vi "Theme Definer UI.vi"() -> ()   [LabVIEW 2021]
doc: "This VI provides a user interface for creating theme style files to output\n\n<b>Code Developed By:</b> +\nDaniel Coons +\nhttps://github.com/danielcoons/tsc-pop-up"
uses:
  Theme/Dialog colors--typedef.ctl
  Theme/Button colors--typedef.ctl
  Theme/message box--typdef.ctl
  <vilib>/picture/picture.llb/imagedata.ctl
  Theme/Theme.lvclass/Theme.ctl
  Popup/PopUp Theme Global.vi
  Theme/Theme.lvclass
  user32.dll
panel:
  in  "Tab Control":enum32{"style file", "material file"}(tab)
  in  "File (.style)":path
  in  "save":bool
  in  "File (.xml)":path
  in  "Theme":u16(ring) items=["Light Theme", "Light Medium Contrast", "Light High Contrast", "Dark Theme", "Dark Medium Contrast", "Dark High Constrast"]
  out "pop-up header":bool
  out "2D Picture":picture
  in  "OK Button":bool
  out "String":string="message input preview"
  in  "Input-string":string="preview"
  in  "Exit":bool
  out "Header":bool
  in  "input":T1={"Text.Font Name"="Segoe UI", "Text.Font Size"=30, "Color"=6579300, "Text.Justification"=enum."Center", "messge color"={"border"=16777215, "fill"=16777215}}
  in  "message font":T1={"Text.Font Name"="Segoe UI", "Text.Font Size"=30, "Color"=6579300, "Text.Justification"=enum."Center", "messge color"={"border"=15790320, "fill"=16777215}}
  in  "button colors":T2={"false color"={"border"=14869218, "fill"=16777215}, "hover color"={"border"=0, "fill"=0}, "press color"={"border"=6579300, "fill"=6579300}, "Boolean Text"=6579300, "Text.Font Name"="Segoe UI", "Text.Font Size"=20, "Bold?"=TRUE, "Itallic?"=FALSE}
  in  "dialog colors":T3={"Header"=11579568, "Background"=15790320, "Picture Background"=16777216}
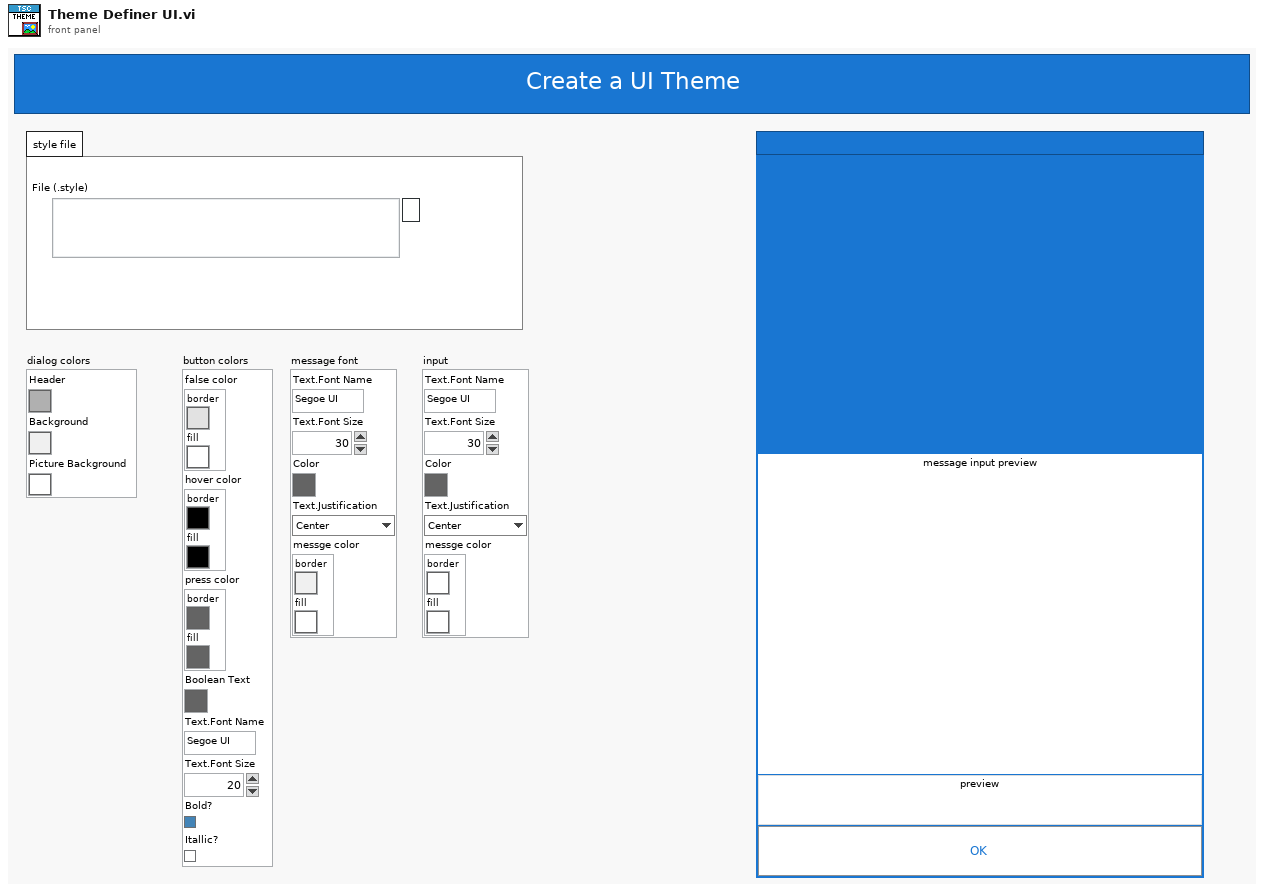
[diagram p1: front panel]
types:
  T1 = typedef "Theme.lvclass/message box--typdef.ctl" = cluster{"Text.Font Name":string, "Text.Font Size":u32, "Color":u32, "Text.Justification":enum16{"Left", "Center", "Right"}, "messge color":cluster{"border":u32, "fill":u32}}
  T2 = typedef "Theme.lvclass/Button colors--typedef.ctl" = cluster{"false color":cluster{"border":u32, "fill":u32}, "hover color":cluster{"border":u32, "fill":u32}, "press color":cluster{"border":u32, "fill":u32}, "Boolean Text":u32, "Text.Font Name":string, "Text.Font Size":u32, "Bold?":bool, "Itallic?":bool}
  T3 = typedef "Theme.lvclass/Dialog colors--typedef.ctl" = cluster{"Header":u32, "Background":u32, "Picture Background":u32}
  T4 = typedef "imagedata.ctl" = cluster{"image type":i32, "image depth":i32, "image":u8[], "mask":u8[], "colors":u32[], "Rectangle":cluster{"left":i16, "top":i16, "right":i16, "bottom":i16}}
  T5 = cluster{"left":i16, "top":i16, "right":i16, "bottom":i16}
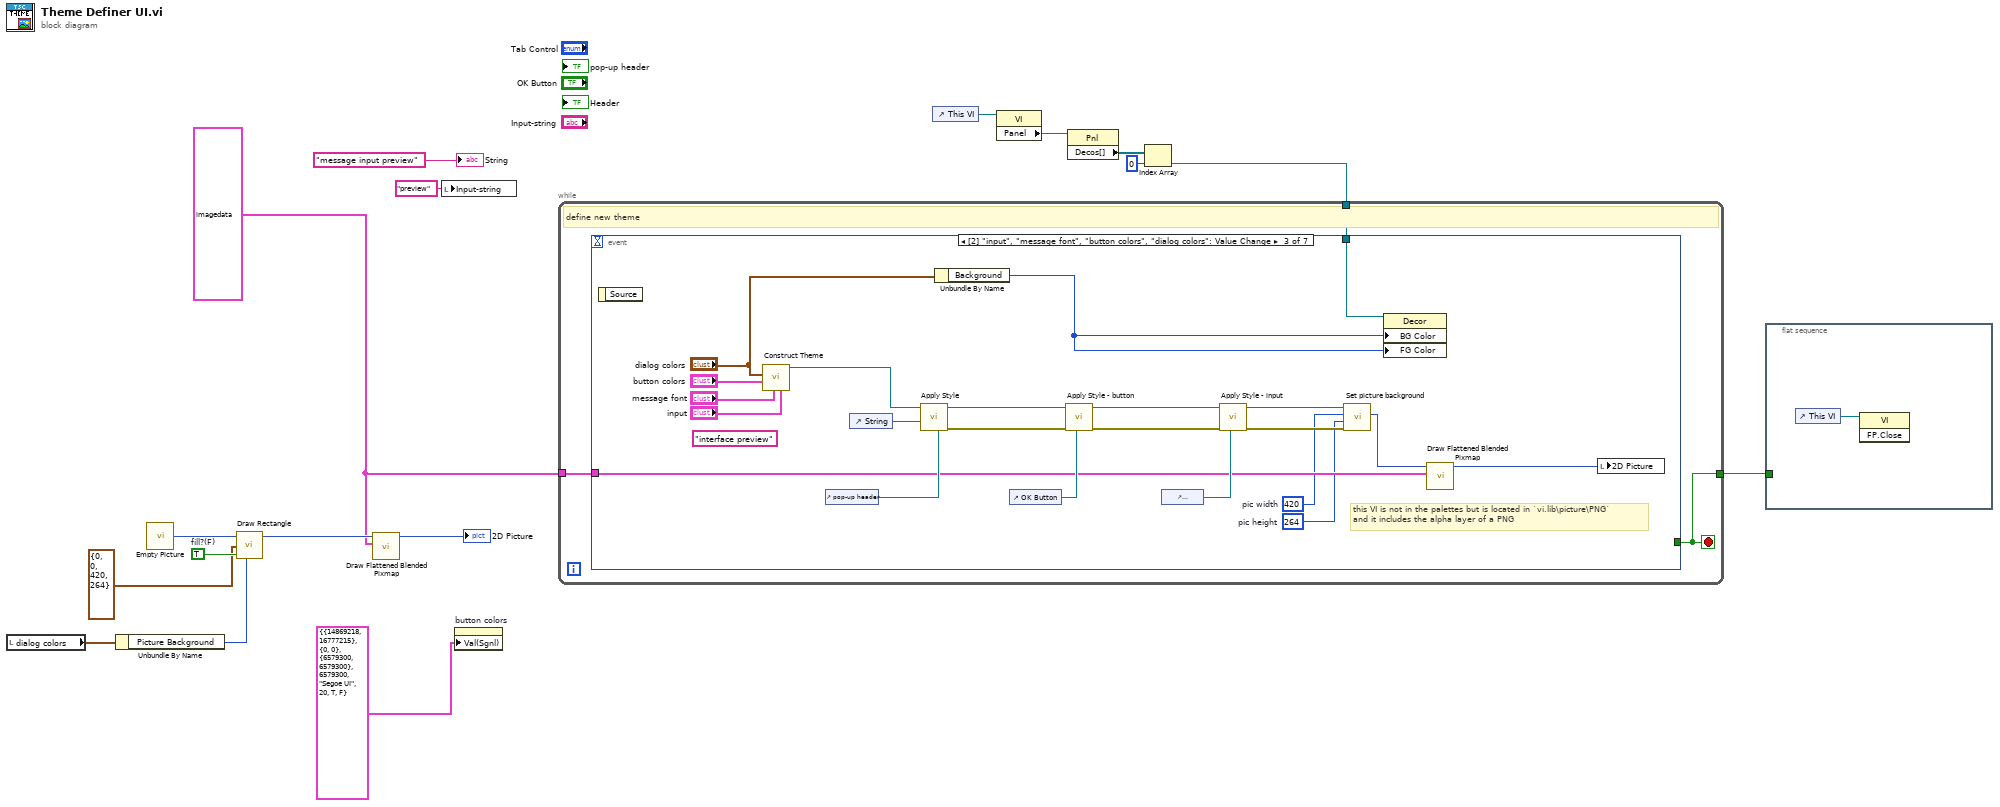
[diagram p0: block diagram]
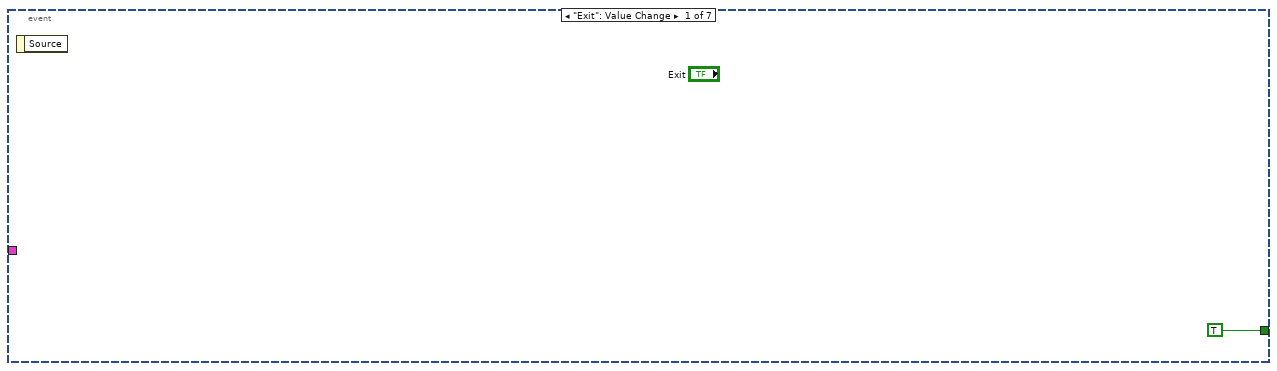
[diagram p2: hidden frame]
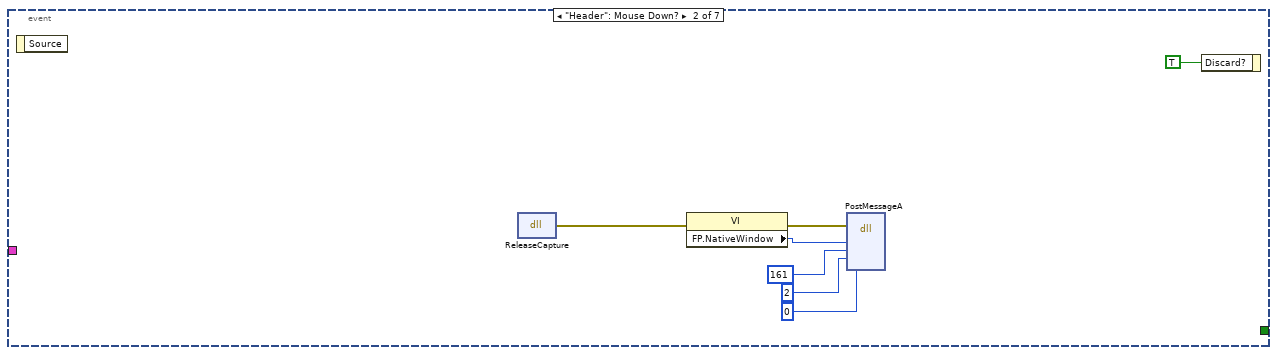
[diagram p3: hidden frame]
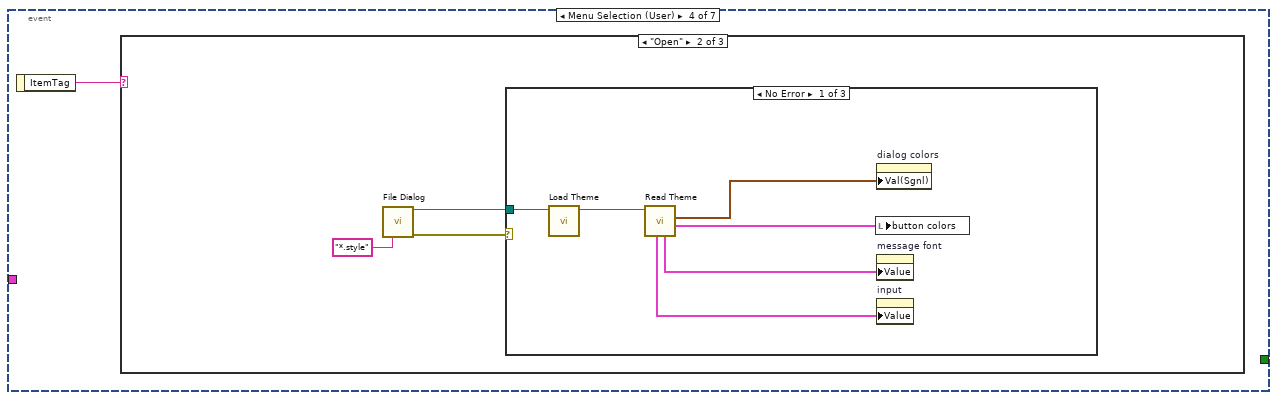
[diagram p4: hidden frame]
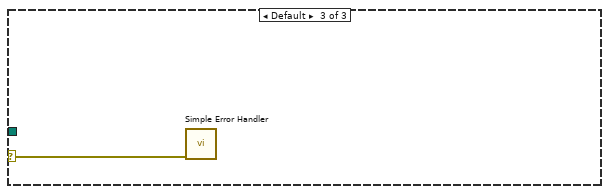
[diagram p7: hidden frame]
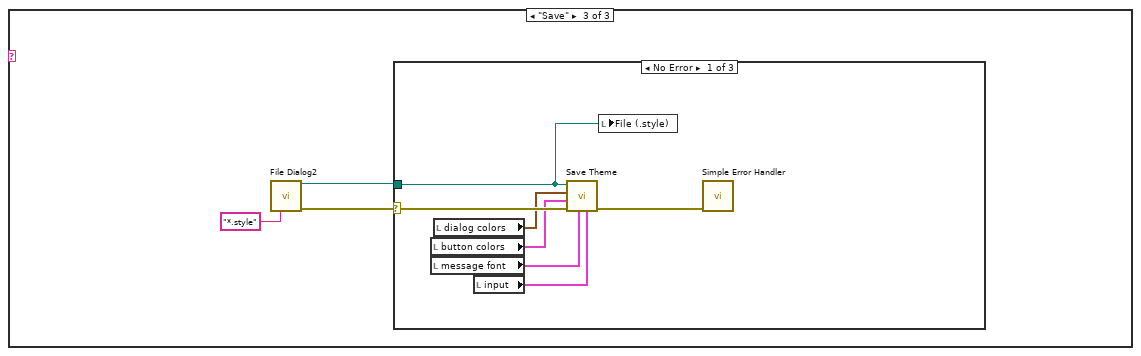
[diagram p8: hidden frame]
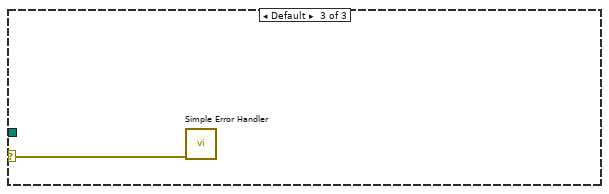
[diagram p10: hidden frame]
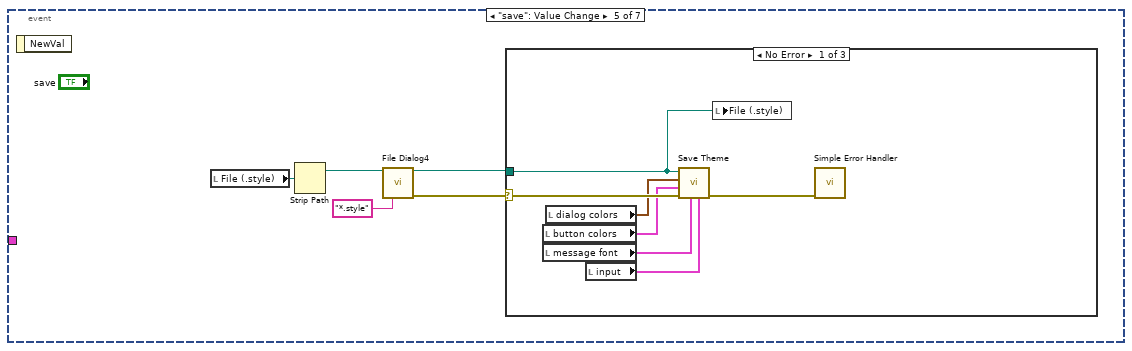
[diagram p11: hidden frame]
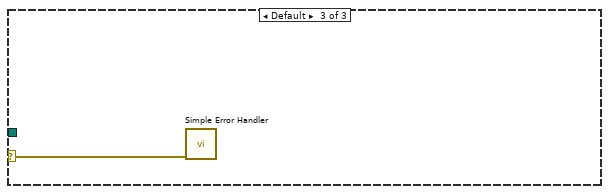
[diagram p13: hidden frame]
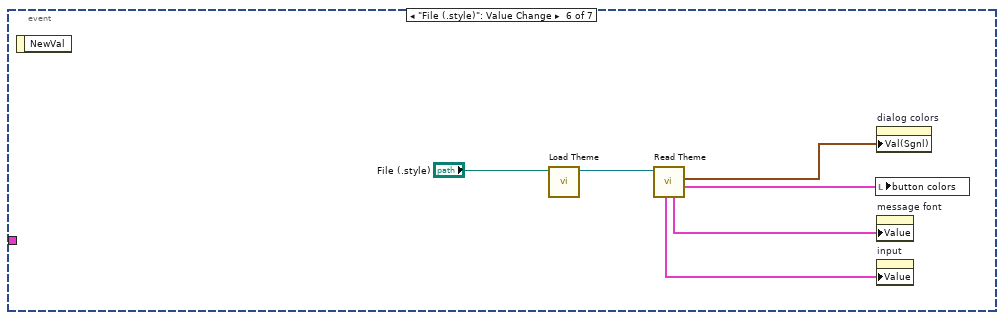
[diagram p14: hidden frame]
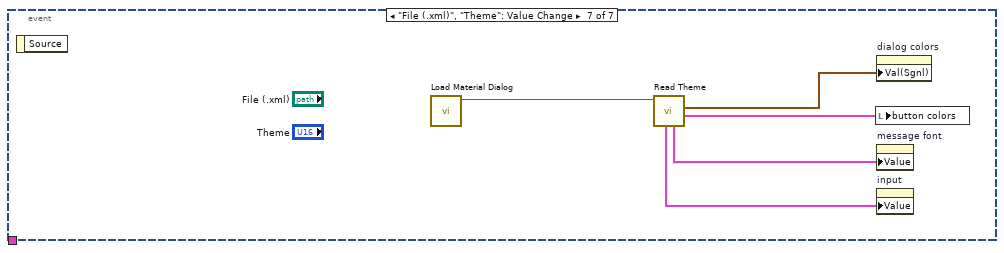
[diagram p15: hidden frame]
diagram:
  w1 = T4 {"image type"=0, "image depth"=32, "image"=array[443520 elements], "mask"=array[14256 elements], "colors"=[], "Rectangle"={"left"=0, "top"=0, "right"=420, "bottom"=264}} ("image data")
  w9 = TRUE  # fill?(F)
  n1 = local read "dialog colors"() -> (w6:T3)
  n2 = Unbundle By Name(w6) -> ("Picture Background"=w3:u32)
  n3 = call "Empty Picture"() -> ("empty picture"=w8:picture)
  n4 = call <vilib>:"Draw Rectangle.vi"("picture"=w8, "rect"=T5 {"left"=0, "top"=0, "right"=420, "bottom"=264}, "fill?(F)"=w9, "color(black)"=w3) -> ("new picture"=w4:picture)  [unwired: 5 in]
  n5 = call <vilib>:"Draw Flattened Blended Pixmap.vi"("image data"=w1, "picture"=w4) -> ("new picture"=→"2D Picture":picture)  [unwired: 6 in, 1 out]
  n6 = local write "Input-string"("preview" ("Input")) -> ()
  n7 = property on="button colors" class="Clust (strict)"("Val(Sgnl)"=T2 {"false color"={"border"=14869218, "fill"=16777215}, "hover color"={"border"=0, "fill"=0}, "press color"={"border"=6579300, "fill"=6579300}, "Boolean Text"=6579300, "Text.Font Name"="Segoe UI", "Text.Font Size"=20, "Bold?"=TRUE, "Itallic?"=FALSE} ("Value (Signaling)")) -> ()  [unwired: 2 in, 2 out]
  n8 = control-ref of="This VI"() -> (w16:refnum<vi>)
  n9 = property class="VI"(reference=w16) -> ("Panel"=w15:refnum<vi>)  [unwired: 1 in, 2 out]
  n10 = property class="Pnl"(reference=w15) -> ("Decos[]"=w14:refnum<vi>[])  [unwired: 1 in, 2 out]
  n11 = Index Array(array=w14, index=0) -> (element=w13:refnum<vi>)
  n12 = while {
    tunnel: w1 -> [w20]
    tunnel: w13 -> [w19]
    tunnel: [w18] -> w10
    stop <- w18 stop-if-true
    # "define new theme"
    n13 = event shown="[2] \"input\", \"message font\", \"button colors\", \"dialog colors\": Value Change" {
      selector: _ -> [_ _ _ _ _ _ _]
      dyn-events: _ -> [_ _ _ _ _ _ _]
      timeout: _ -> [_ _ _ _ _ _ _]
      tunnel: [TRUE _ _ _ _ _ _] -> w18
      tunnel: w20 -> [_ _ w39 _ _ _ _]
      tunnel: w19 -> [_ _ w37 _ _ _ _]
      event "Exit": Value Change {
        n14 = event-data() -> ()  [unwired: 1 in, 1 out]
      }
      event "Header": Mouse Down? {
        n15 = event-data() -> ()  [unwired: 1 in, 1 out]
        n16 = dll-call lib="user32.dll" fn="ReleaseCapture"() -> (error out=w24:errorcluster)  [unwired: 4 in, 1 out]
        n17 = property class="VI"(error in=w24) -> (error out=w23:errorcluster, "FP.NativeWindow"=w22:u64)  [unwired: 1 in, 1 out]
        n18 = dll-call lib="user32.dll" fn="PostMessageA"(error in=w23, "hWnd"=w22, "Msg"=161, "wParam"=2, "lParam"=0) -> ()  [unwired: 7 in, 2 out]
        n19 = event-data("Discard?"=TRUE) -> ()  [unwired: 1 in, 1 out]
      }
      event Value Change {
        w29 = i16 264  # pic height
        w30 = i16 420  # pic width
        (unwired) "interface preview" ("Message")
        # "this VI is not in the palettes but is located in `vi.lib\\picture\\PNG`\nand it includes the alpha layer of a PNG"
        n20 = event-data() -> ()  [unwired: 1 in, 1 out]
        n21 = call "Construct Theme.vi"("input"="input", "message font"="message font", "button colors"="button colors", "dialog colors"="dialog colors") -> ("Theme out"=w35:refnum<class "Theme.lvclass">)  [unwired: 6 in, 1 out]
        n22 = control-ref of="pop-up header"() -> (w44:refnum<vi>)
        n23 = control-ref of="String"() -> (w42:refnum<vi>)
        n24 = call "Apply Style.vi"("header ref"=w44, "message ref"=w42, "Theme in"=w35) -> ("error out"=w43:errorcluster, "Theme out"=w47:refnum<class "Theme.lvclass">)  [unwired: 7 in]
        n25 = Unbundle By Name("dialog colors") -> ("Background"=w36:u32)
        n26 = control-ref of="OK Button"() -> (w48:refnum<vi>)
        n27 = call "Apply Style - button.vi"("button ref"=w48, "error in"=w43, "Theme in"=w47) -> ("error out"=w45:errorcluster, "Theme out"=w46:refnum<class "Theme.lvclass">)  [unwired: 7 in]
        n28 = control-ref of="Input-string"() -> (w49:refnum<vi>)
        n29 = call "Apply Style - input.vi"("input ref"=w49, "error in (no error)"=w45, "Theme in"=w46) -> ("error out"=w31:errorcluster, "Theme out"=w41:refnum<class "Theme.lvclass">)  [unwired: 7 in]
        n30 = call "Set picture background.vi"("error in"=w31, "pic height"=w29, "pic width"=w30, "Theme in"=w41) -> ("background"=w40:picture)  [unwired: 5 in, 2 out]
        n31 = property class="Decor"(reference=w37, "BG Color"=w36, "FG Color"=w36) -> ()  [unwired: 1 in, 2 out]
        n32 = call <vilib>:"Draw Flattened Blended Pixmap.vi"("image data"=w39, "picture"=w40) -> ("new picture"=w38:picture)  [unwired: 6 in, 1 out]
        n33 = local write "2D Picture"(w38) -> ()
      }
      event Menu Selection (User) {
        n34 = event-data() -> ("ItemTag"=w51:string)  [unwired: 1 in]
        n35 = case shown="\"Open\"" w51 {
          frame Default {
          }
          frame "Open" {
            n36 = call "File Dialog"("pattern (all files)"="*.style") -> ("selected path"=w52:path, "error out"=w53:errorcluster)  [unwired: 11 in, 2 out]
            n37 = case shown="No Error" w53 {
              selector: w53 -> [_ _ w61]
              tunnel: w52 -> [w60 _ _]
              frame No Error {
                n38 = call "Load Theme.vi"("File Path"=w60) -> ("Theme"=w59:refnum<class "Theme.lvclass">)  [unwired: 9 in, 1 out]
                n39 = call "Read Theme.vi"("Theme in"=w59) -> ("button colors"=w57:T2, "dialog colors"=w58:T3, "message font"=w56:T1, "input"=w55:T1)  [unwired: 6 in, 1 out]
                n40 = local write "button colors"(w57) -> ()
                n41 = property on="dialog colors" class="Clust (strict)"("Val(Sgnl)"=w58) -> ()  [unwired: 2 in, 2 out]
                n42 = property on="message font" class="Clust (strict)"("Value"=w56) -> ()  [unwired: 2 in, 2 out]
                n43 = property on="input" class="Clust (strict)"("Value"=w55) -> ()  [unwired: 2 in, 2 out]
              }
              frame Error {
              }
              frame Default {
                n44 = call <vilib>:"Simple Error Handler.vi"("error in (no error)"=w61) -> ()  [unwired: 4 in, 5 out]
              }
            }
          }
          frame "Save" {
            n45 = call "File Dialog2"("pattern (all files)"="*.style") -> ("selected path"=w62:path, "error out"=w63:errorcluster)  [unwired: 11 in, 2 out]
            n46 = case shown="No Error" w63 {
              selector: w63 -> [w71 _ w72]
              tunnel: w62 -> [w65 _ _]
              frame No Error {
                n47 = local read "button colors"() -> (w69:T2)
                n48 = local read "message font"() -> (w68:T1)
                n49 = local read "dialog colors"() -> (w70:T3)
                n50 = local read "input"() -> (w67:T1)
                n51 = call "Save Theme.vi"("input"=w67, "message font"=w68, "error in"=w71, "button colors"=w69, "dialog colors"=w70, "File"=w65) -> ("error out"=w66:errorcluster)  [unwired: 5 in]
                n52 = local write "File (.style)"(w65) -> ()
                n53 = call <vilib>:"Simple Error Handler.vi"("error in (no error)"=w66) -> ()  [unwired: 4 in, 5 out]
              }
              frame Error {
              }
              frame Default {
                n54 = call <vilib>:"Simple Error Handler.vi"("error in (no error)"=w72) -> ()  [unwired: 4 in, 5 out]
              }
            }
          }
        }
      }
      event "save": Value Change {
        n55 = event-data() -> ()  [unwired: 1 in, 1 out]
        n56 = local read "File (.style)"() -> (w74:path)
        n57 = Strip Path(path=w74) -> (stripped path=w73:path)  [unwired: 1 out]
        n58 = call "File Dialog4"("start path"=w73, "pattern (all files)"="*.style") -> ("selected path"=w75:path, "error out"=w76:errorcluster)  [unwired: 10 in, 2 out]
        n59 = case shown="No Error" w76 {
          selector: w76 -> [w84 _ w85]
          tunnel: w75 -> [w78 _ _]
          frame No Error {
            n60 = local read "button colors"() -> (w82:T2)
            n61 = local read "message font"() -> (w81:T1)
            n62 = local read "dialog colors"() -> (w83:T3)
            n63 = local read "input"() -> (w80:T1)
            n64 = call "Save Theme.vi"("input"=w80, "message font"=w81, "error in"=w84, "button colors"=w82, "dialog colors"=w83, "File"=w78) -> ("error out"=w79:errorcluster)  [unwired: 5 in]
            n65 = local write "File (.style)"(w78) -> ()
            n66 = call <vilib>:"Simple Error Handler.vi"("error in (no error)"=w79) -> ()  [unwired: 4 in, 5 out]
          }
          frame Error {
          }
          frame Default {
            n67 = call <vilib>:"Simple Error Handler.vi"("error in (no error)"=w85) -> ()  [unwired: 4 in, 5 out]
          }
        }
      }
      event "File (.style)": Value Change {
        n68 = event-data() -> ()  [unwired: 1 in, 1 out]
        n69 = call "Load Theme.vi"("File Path"="File (.style)") -> ("Theme"=w90:refnum<class "Theme.lvclass">)  [unwired: 9 in, 1 out]
        n70 = call "Read Theme.vi"("Theme in"=w90) -> ("button colors"=w88:T2, "dialog colors"=w89:T3, "message font"=w86:T1, "input"=w87:T1)  [unwired: 6 in, 1 out]
        n71 = local write "button colors"(w88) -> ()
        n72 = property on="dialog colors" class="Clust (strict)"("Val(Sgnl)"=w89) -> ()  [unwired: 2 in, 2 out]
        n73 = property on="message font" class="Clust (strict)"("Value"=w86) -> ()  [unwired: 2 in, 2 out]
        n74 = property on="input" class="Clust (strict)"("Value"=w87) -> ()  [unwired: 2 in, 2 out]
      }
      event "File (.xml)", "Theme": Value Change {
        n75 = event-data() -> ()  [unwired: 1 in, 1 out]
        n76 = call "Load Material Dialog.vi"() -> ("Theme Obj"=w96:refnum<class "Theme.lvclass">)  [unwired: 10 in, 1 out]
        n77 = call "Read Theme.vi"("Theme in"=w96) -> ("button colors"=w94:T2, "dialog colors"=w95:T3, "message font"=w92:T1, "input"=w93:T1)  [unwired: 6 in, 1 out]
        n78 = local write "button colors"(w94) -> ()
        n79 = property on="dialog colors" class="Clust (strict)"("Val(Sgnl)"=w95) -> ()  [unwired: 2 in, 2 out]
        n80 = property on="message font" class="Clust (strict)"("Value"=w92) -> ()  [unwired: 2 in, 2 out]
        n81 = property on="input" class="Clust (strict)"("Value"=w93) -> ()  [unwired: 2 in, 2 out]
      }
    }
  }
  n82 = flat-sequence {
    tunnel: w10 -> [_]
    frame #0 {
      n83 = control-ref of="This VI"() -> (w97:refnum<vi>)
      n84 = invoke class="VI" method="FP.Close"(reference=w97) -> ()  [unwired: 2 in, 3 out]
    }
  }
  "String" <- "message input preview" ("String")
